vi "JSON Array to LabVIEW Array Base Type.vi"(8 "error in (no error)":errorcluster, 10 "Type of Array In":T1=enum."Unknown", 11 "JSON Array In":variant) -> (0 "error out":errorcluster, 3 "LabVIEW Array Base Type Out":variant)   [LabVIEW 2013, in "i3-json.lvlib"]
doc: "Attempts to write the data from the JSON Array to the LabVIEW Array control specified."
uses:
  i3-json.lvlib
  JSON Types/JSON Type.ctl
  Error/Invalid Type Error.vi
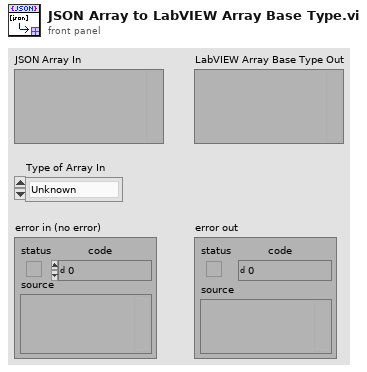
[diagram p1: front panel]
types:
  T1 = typedef "i3-json.lvlib/JSON Type.ctl" = enum8{"JSON Compatible", "JSON Array", "JSON Object", "JSON Null", "Double", "String", "Boolean", "Unknown"}
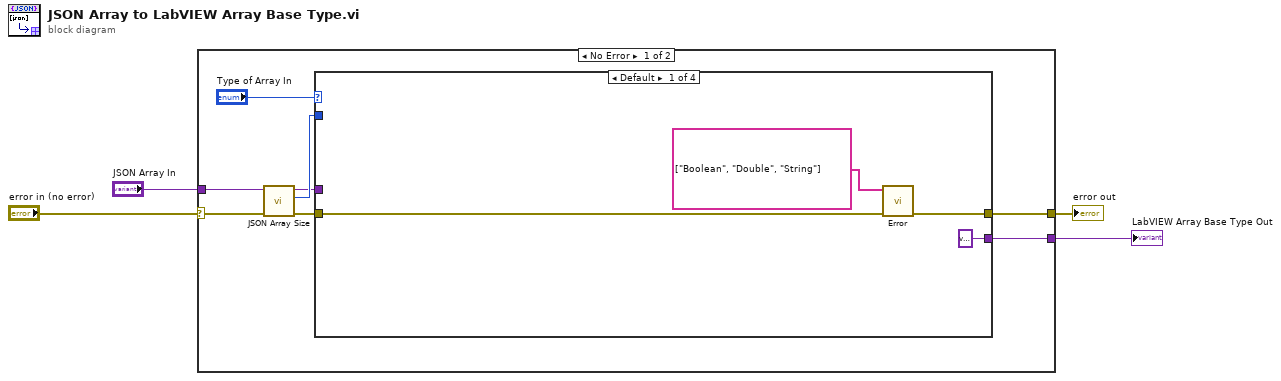
[diagram p0: block diagram]
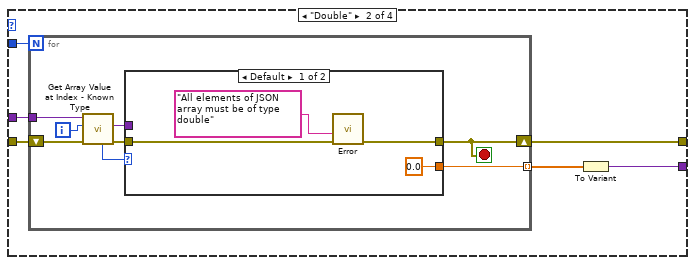
[diagram p2: hidden frame]
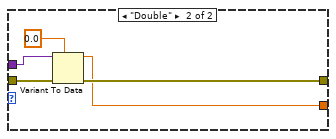
[diagram p3: hidden frame]
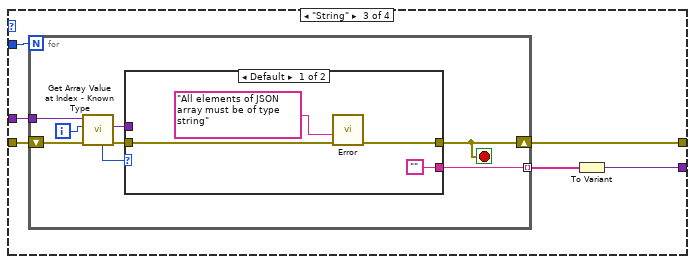
[diagram p4: hidden frame]
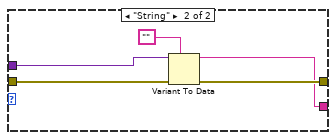
[diagram p5: hidden frame]
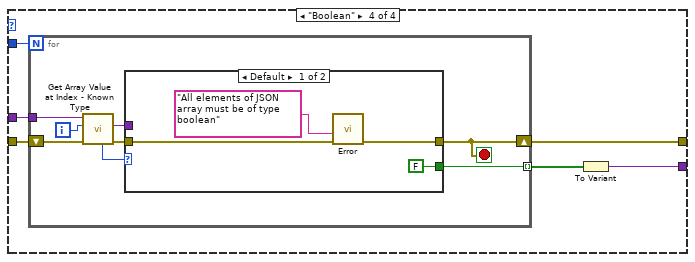
[diagram p6: hidden frame]
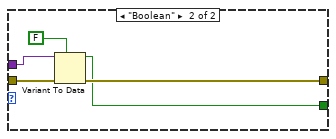
[diagram p7: hidden frame]
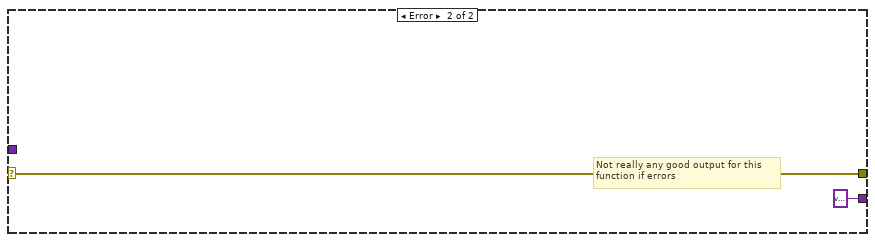
[diagram p8: hidden frame]
diagram:
  n1 = case shown="No Error" "error in (no error)" {
    selector: "error in (no error)" -> [w6 w86]
    tunnel: "JSON Array In" -> [w5 _]
    tunnel: [w12 w86] -> w2
    tunnel: [w11 variant ("Variant")] -> w1
    frame No Error {
      n2 = call "JSON Array Size.vi"("error in (no error)"=w6, "JSON Tree In (JSON Array)"=w5) -> ("error out"=w9:errorcluster, "Array Size"=w10:i32, "JSON Tree Passthrough (JSON Array)"=w8:variant)  [unwired: 7 in]
      n3 = case shown="Default" "Type of Array In" {
        tunnel: w10 -> [_ w22 w45 w68]
        tunnel: w9 -> [w14 w21 w44 w67]
        tunnel: w8 -> [_ w20 w43 w66]
        tunnel: [w13 w19 w42 w65] -> w12
        tunnel: [variant ("Variant") w18 w41 w64] -> w11
        frame Default {
          n4 = call-poly "Error.vi"("error in (no error)"=w14, "Valid Types"=string[] ["Boolean", "Double", "String"]) -> ("error out"=w13:errorcluster)  [unwired: 9 in]
        }
        frame "Double" {
          n5 = for {
            N: w22 -> [_]
            tunnel: w20 -> [w30]
            tunnel: [w24] -> w17 mode=indexing
            shift-right: [w23] -> w19
            shift-left: w21 -> [w29]
            i -> [w28]
            stop <- w23 stop-if-true
            n6 = call "Get Array Value at Index - Known Type.vi"("error in (no error)"=w29, "Index"=w28, "JSON Tree In (JSON Array)"=w30) -> ("error out"=w25:errorcluster, "Value"=w26:variant, "JSON Type"=w27:T1)  [unwired: 3 in, 3 out]
            n7 = case shown="Default" w27 {
              tunnel: w26 -> [_ w38]
              tunnel: w25 -> [w31 w39]
              tunnel: [w33 w36] -> w23
              tunnel: [0.0 w35] -> w24
              frame Default {
                n8 = call-poly "Error.vi"("error in (no error)"=w31, "additional info"="All elements of JSON array must be of type double" ("source")) -> ("error out"=w33:errorcluster)  [unwired: 9 in]
              }
              frame "Double" {
                n9 = Variant To Data(error in=w39, type=0.0, Variant=w38) -> (data=w35:dbl, error out=w36:errorcluster)
              }
            }
          }
          n10 = To Variant(anything=w17) -> (Variant=w18:variant)
        }
        frame "String" {
          n11 = for {
            N: w45 -> [_]
            tunnel: w43 -> [w53]
            tunnel: [w47] -> w40 mode=indexing
            shift-right: [w46] -> w42
            shift-left: w44 -> [w52]
            i -> [w51]
            stop <- w46 stop-if-true
            n12 = call "Get Array Value at Index - Known Type.vi"("error in (no error)"=w52, "Index"=w51, "JSON Tree In (JSON Array)"=w53) -> ("error out"=w48:errorcluster, "Value"=w49:variant, "JSON Type"=w50:T1)  [unwired: 3 in, 3 out]
            n13 = case shown="Default" w50 {
              tunnel: w49 -> [_ w61]
              tunnel: w48 -> [w54 w62]
              tunnel: [w55 w60] -> w46
              tunnel: ["" w59] -> w47
              frame Default {
                n14 = call-poly "Error.vi"("error in (no error)"=w54, "additional info"="All elements of JSON array must be of type string" ("source")) -> ("error out"=w55:errorcluster)  [unwired: 9 in]
              }
              frame "String" {
                n15 = Variant To Data(error in=w62, type="", Variant=w61) -> (data=w59:string, error out=w60:errorcluster)
              }
            }
          }
          n16 = To Variant(anything=w40) -> (Variant=w41:variant)
        }
        frame "Boolean" {
          n17 = for {
            N: w68 -> [_]
            tunnel: w66 -> [w76]
            tunnel: [w70] -> w63 mode=indexing
            shift-right: [w69] -> w65
            shift-left: w67 -> [w75]
            i -> [w74]
            stop <- w69 stop-if-true
            n18 = call "Get Array Value at Index - Known Type.vi"("error in (no error)"=w75, "Index"=w74, "JSON Tree In (JSON Array)"=w76) -> ("error out"=w71:errorcluster, "Value"=w72:variant, "JSON Type"=w73:T1)  [unwired: 3 in, 3 out]
            n19 = case shown="Default" w73 {
              tunnel: w72 -> [_ w84]
              tunnel: w71 -> [w77 w85]
              tunnel: [w78 w83] -> w69
              tunnel: [FALSE w82] -> w70
              frame Default {
                n20 = call-poly "Error.vi"("error in (no error)"=w77, "additional info"="All elements of JSON array must be of type boolean" ("source")) -> ("error out"=w78:errorcluster)  [unwired: 9 in]
              }
              frame "Boolean" {
                n21 = Variant To Data(error in=w85, type=FALSE, Variant=w84) -> (data=w82:bool, error out=w83:errorcluster)
              }
            }
          }
          n22 = To Variant(anything=w63) -> (Variant=w64:variant)
        }
      }
    }
    frame Error {
      # "Not really any good output for this\nfunction if errors"
    }
  }
  "LabVIEW Array Base Type Out" <- w1
  "error out" <- w2
